vi "Vision Processing.vi"(4 "error in (no error)":errorcluster, 5 "Camera Type":enum16{"206", "1011"}(ring)=enum."1011", 6 "Camera Name":string="Camera") -> ()   [LabVIEW 2012]
uses:
  Robot Global Data.vi
  <vilib>/vision/NI_Vision_Development_Module.lvlib
panel:
  in  "Color Enabled":bool
  in  "Range":cluster{"Lower value":sgl, "Upper value":sgl}={"Lower value"=247.60869, "Upper value"=255.0} {"Lower value" scale=0.0..255.0; "Upper value" scale=0.0..255.0}
  out "Target Info":cluster{"X":dbl, "Y":dbl, "Distance (ft)":dbl}
  in  "Enable Vision":bool=TRUE
  in  "View":bool
  out "Target Info":T1(array[cluster])
  in  "Area Size Limit %":dbl=0.5
  in  "Particle Count Limit":i32=8
  in  "Score Limits":T2={"Rect Coverage"=60.0, "X Edge Strength"=40.0, "Y Edge Strength"=60.0, "Center"=75.0, "Outer"=75.0}
  in  "View":bool
  out "Processed Image":T3(plugin-control)
  out "Original Image":T3(plugin-control)
  # "Instructions:\nProcessing the reflective tape that is illuminated by a ring light can be based\non color or light intensity.\nParticles within the image are scored by rectangle coverage, aspect ratio, and\nfor being hollow with a bold edge. A particle is considered a target if all scores\nare above the score limits. Particles can be annotated -- surrounded by\na rectangle and scores drawn to the left .\nTo control the number of particles being scored, use the count limit and the size\nlimit."
  # "To debug, Enable using the View button.\nFor color processing, you can click in the image to select the color for processing."
  # "Enable by clicking the View button.\nGreen scores are above the limit, orange are below. Inner/outer rect\nindicates all passed."
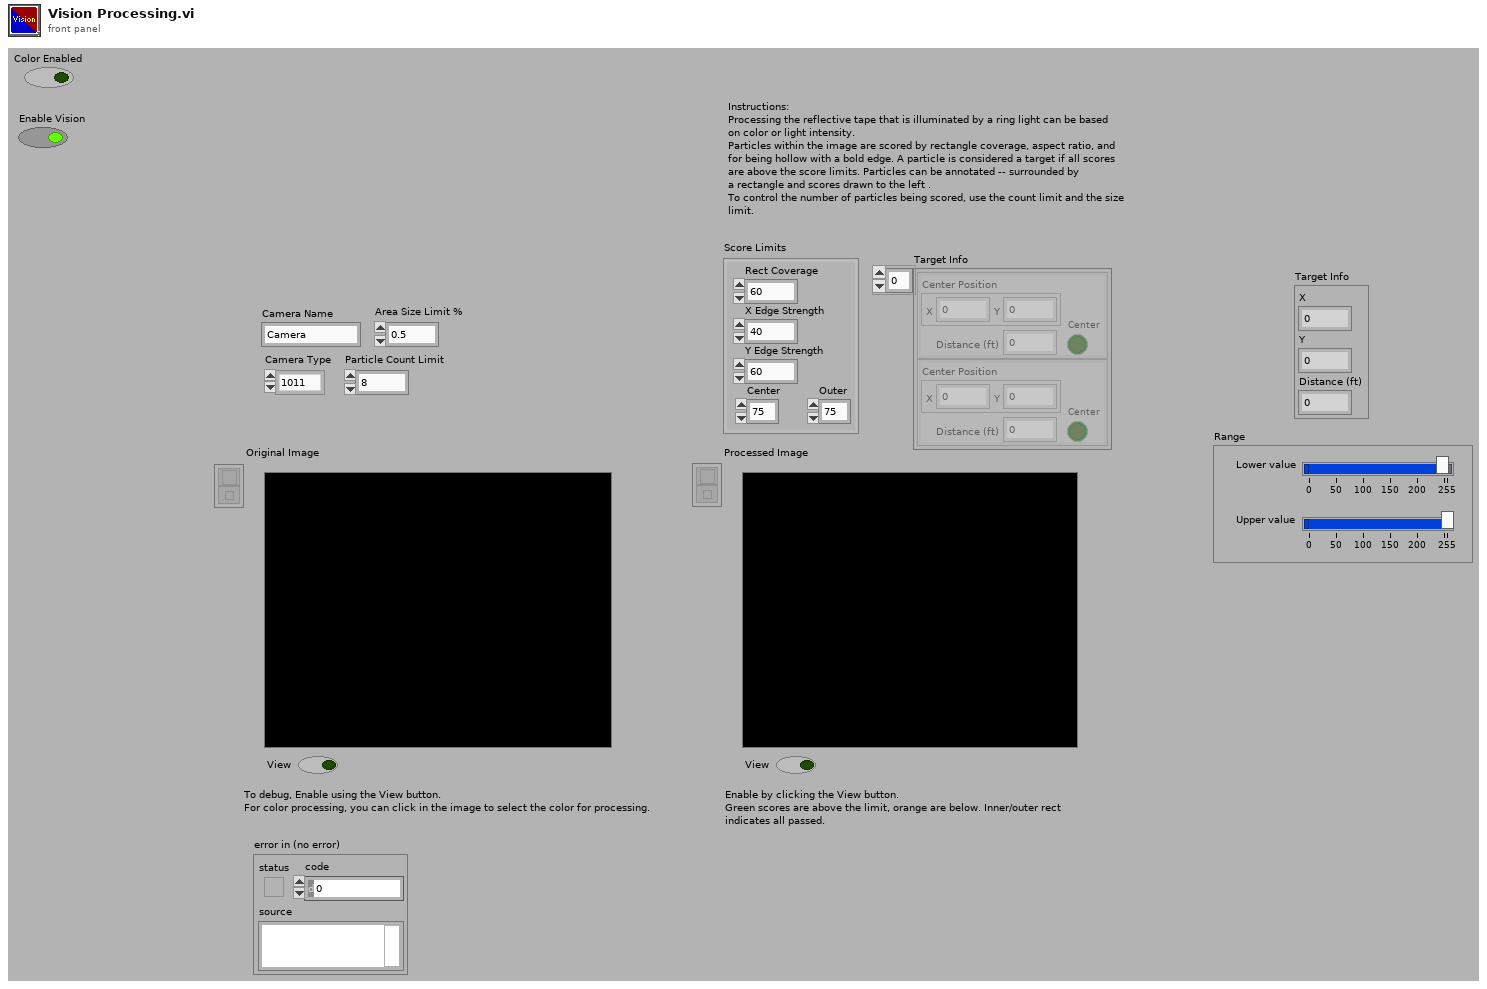
[diagram p1: front panel]
types:
  T1 = cluster{"Center Position":cluster{"X":dbl, "Y":dbl}, "Distance (ft)":dbl, "Center":bool}[]
  T2 = cluster{"Rect Coverage":dbl, "X Edge Strength":dbl, "Y Edge Strength":dbl, "Center":dbl, "Outer":dbl}
  T3 = typedef "IMAQ Image.ctl" = refnum<image>
  T4 = typedef "Image Type" = u32
  T5 = typedef "WPI_CameraDevRef.ctl" = cluster{"Camera Address":string, "CameraStatus":errorcluster, "Acquire Image Notifier":refnum<notifier>}
  T6 = cluster{"Position":cluster{"X":dbl, "Y":dbl}, "Distance (ft)":dbl, "Center":bool}[]
  T7 = typedef "WPI_CameraImageSize.ctl" = enum16{"640x480", "320x240", "160x120"}
  T8 = cluster{cluster{"Left":dbl, "Top":dbl, "Right":dbl, "Bottom":dbl}, "Scores":dbl[], cluster{"Long":dbl, "Short":dbl}}[]
  T9 = cluster{"Target Center (-1 to 1)":cluster{"X":dbl, "Y":dbl}, "Distance (ft)":dbl, "Center Target":bool}
  T10 = cluster{"Target Center (-1 to 1)":cluster{"X":dbl, "Y":dbl}, "Distance (ft)":dbl, "Center Target":bool}[]
  T11 = cluster{"Left":dbl, "Top":dbl, "Right":dbl, "Bottom":dbl}
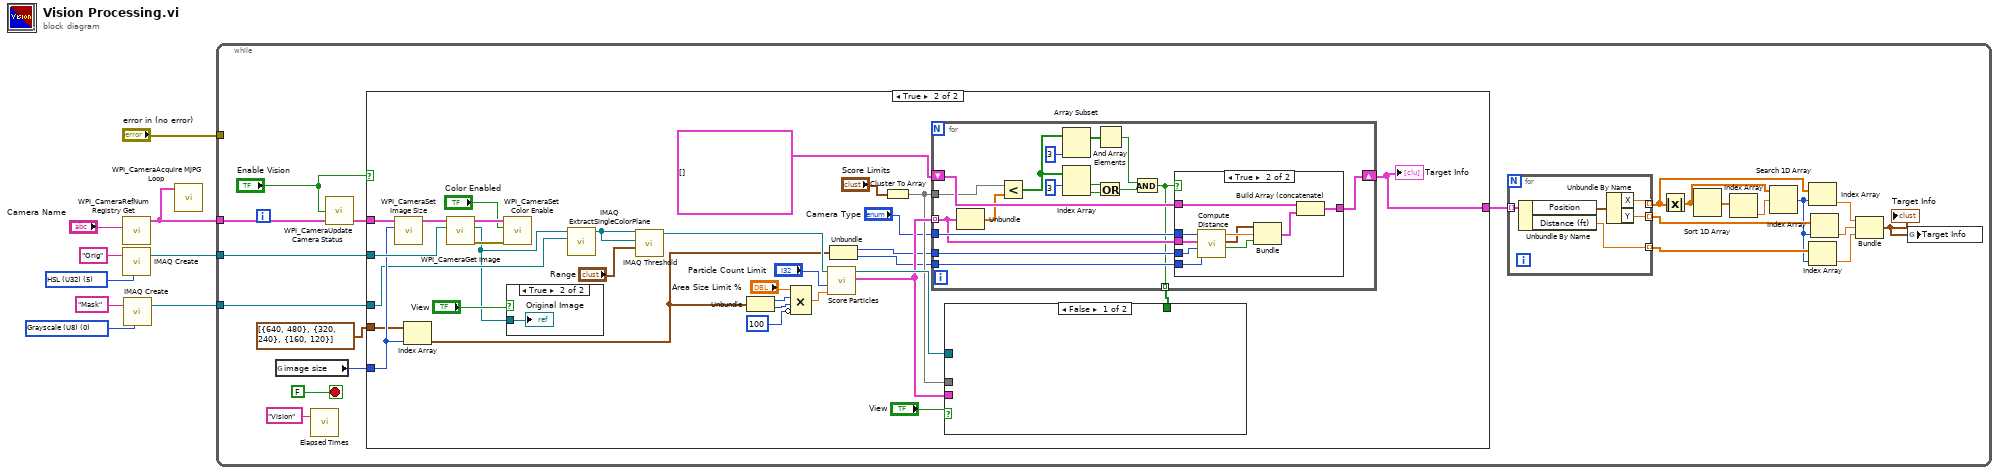
[diagram p0: block diagram]
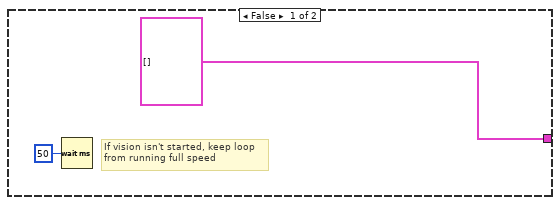
[diagram p2: hidden frame]
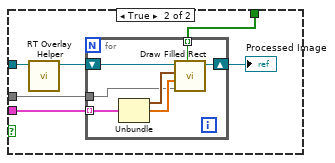
[diagram p4: hidden frame]
diagram:
  w3 = T4 0 items=["Grayscale (U8)", "Grayscale (I16)", "Grayscale (SGL)", "Complex (CSG)", "RGB (U32)", "HSL (U32)", "RGB (U64)", "Grayscale (U16)"] ("Image Type")
  w8 = T4 5 items=["Grayscale (U8)", "Grayscale (I16)", "Grayscale (SGL)", "Complex (CSG)", "RGB (U32)", "HSL (U32)", "RGB (U64)", "Grayscale (U16)"] ("Image Type")
  n1 = call <vilib>:"WPI_CameraRefNum Registry Get.vi"("refnum name"="Camera Name") -> ("CameraDevRef"=w5:T5)  [unwired: 9 in, 1 out]
  n2 = call "IMAQ Create"("Image Name"="Orig", "Image Type"=w8) -> ("New Image"=w7:T3)  [unwired: 2 in, 2 out]
  n3 = call "IMAQ Create"("Image Name"="Mask", "Image Type"=w3) -> ("New Image"=w1:T3)  [unwired: 2 in, 2 out]
  n4 = call <vilib>:"WPI_CameraAcquire MJPG Loop.vi"("CameraDevRef"=w5) -> ()  [unwired: 11 in]
  n5 = while {
    tunnel: w7 -> [w29]
    tunnel: w5 -> [w28]
    tunnel: "error in (no error)" -> [_]
    tunnel: w1 -> [w25]
    stop <- FALSE stop-if-true
    n6 = global read "Robot Global Data.vi" "image size"() -> (w26:T7)
    n7 = call "Elapsed Times.vi"("Call Name"="Vision") -> ()  [unwired: 2 in, 1 out]
    n8 = call <vilib>:"WPI_CameraUpdate Camera Status.vi"("CameraDevRef In"=w28, "Enable Vision"="Enable Vision") -> ("CameraDevRef Out"=w27:T5)  [unwired: 3 in]
    n9 = case shown="True" "Enable Vision" {
      tunnel: w29 -> [_ w64]
      tunnel: w27 -> [_ w60]
      tunnel: w26 -> [_ w57]
      tunnel: w25 -> [_ w53]
      tunnel: cluster{i32, i32}[] [{640, 480}, {320, 240}, {160, 120}] -> [_ w56]
      tunnel: [T6 [] w47] -> w21
      frame False {
        # "If vision isn't started, keep loop\nfrom running full speed"
        n10 = Wait (ms)(milliseconds to wait=u32 50) -> ()  [unwired: 1 out]
      }
      frame True {
        n11 = call <vilib>:"WPI_CameraSet Image Size.vi"("Image Size"=w57, "CameraDevRef"=w60) -> ("CameraDevRef Out"=w61:T5)  [unwired: 8 in, 1 out]
        n12 = Index Array(array=w56, index=w57) -> (element=w48:cluster{i32, i32})
        n13 = call <vilib>:"WPI_CameraGet Image.vi"("Image"=w64, "CameraDevRef"=w61) -> ("error out"=w62:errorcluster, "Image Out"=w52:T3, "CameraDevRef Out"=w63:T5)  [unwired: 7 in]
        n14 = call <vilib>:"WPI_CameraSet Color Enable.vi"("error in (no error)"=w62, "Color Enabled"="Color Enabled", "CameraDevRef"=w63) -> ()  [unwired: 7 in, 2 out]
        n15 = case shown="True" "View" {
          tunnel: w52 -> [_ w111]
          frame False {
          }
          frame True {
            "Original Image" <- w111
          }
        }
        n16 = call "IMAQ ExtractSingleColorPlane"("Image Dst"=w53, "Image Src"=w52) -> ("Image Dst Out"=w45:T3)  [unwired: 8 in, 1 out]
        n17 = call "IMAQ Threshold"("Range"="Range", "Image Dst"=w45, "Image Src"=w45) -> ("Image Dst Out"=w58:T3)  [unwired: 3 in, 5 out]
        n18 = Unbundle(w48) -> (w41:i32, w40:i32)
        n19 = Compound Arithmetic op=MULTIPLY("Area Size Limit %", w41, w40, invert 100 ("length")) -> (w38:dbl)
        n20 = call "Score Particles.vi"("Area Size Limit"=w38, "Particle Count Limit"="Particle Count Limit", "Image Refnum in"=w58) -> ("Scored Particle Info"=w67:T8, "Image Refnum out"=w69:T3)  [unwired: 7 in]
        n21 = Unbundle(w48) -> (w55:i32, w54:i32)
        n22 = Cluster To Array(cluster="Score Limits") -> (array=w65:dbl[])
        n23 = for {
          shift-right: [w85] -> w47
          shift-left: T6 [] -> [w86]
          tunnel: w55 -> [w84]
          tunnel: w67 -> [w79] mode=indexing
          tunnel: w65 -> [w81]
          tunnel: "Camera Type" -> [w83]
          tunnel: w54 -> [w80]
          tunnel: [w70] -> w49 mode=indexing
          n24 = Unbundle(w79) -> ("Scores"=w82:dbl[])  [unwired: 2 out]
          n25 = Less?(x=w81, y=w82) -> (x < y?=w71:bool[])
          n26 = Array Subset(array=w71, length=3) -> (w73:bool[])  [unwired: 1 in]
          n27 = Index Array(array=w71, index #1=3 ("length")) -> (element #1=w75:bool, element #2=w76:bool)  [unwired: 1 in]
          n28 = And Array Elements(Boolean array=w73) -> (logical AND=w78:bool)
          n29 = Or(x=w75, y=w76) -> (x .or. y?=w77:bool)
          n30 = And(x=w78, y=w77) -> (x .and. y?=w70:bool)
          n31 = case shown="True" w70 {
            tunnel: w86 -> [w87 w97]
            tunnel: [w87 w96] -> w85
            tunnel: w84 -> [_ w94]
            tunnel: w83 -> [_ w92]
            tunnel: w80 -> [_ w91]
            tunnel: w79 -> [_ w89]
            frame False {
            }
            frame True {
              n32 = call "Compute Distance.vi"("Y Image Resolution"=w91, "X Image Resolution"=w94, "Particle Scores"=w89, "Camera Type"=w92) -> ("Center Target"=w88:bool, "Target Center (-1 to 1)"=w90:cluster{"X":dbl, "Y":dbl}, "Distance (ft)"=w93:dbl)  [unwired: 5 in]
              n33 = Bundle("Target Center (-1 to 1)"=w90, "Distance (ft)"=w93, "Center Target"=w88) -> (w95:T9)  [unwired: 1 in]
              n34 = Build Array (concatenate)(w97, w95) -> (w96:T10)
            }
          }
        }
        "Target Info" <- w47
        n35 = case shown="False" "View" {
          tunnel: w69 -> [_ w100]
          tunnel: w67 -> [_ w102]
          tunnel: w65 -> [_ w101]
          tunnel: w49 -> [_ w98]
          frame False {
          }
          frame True {
            n36 = call "RT Overlay Helper.vi"("Refnum in"=w100) -> ("Refnum out"=w103:T3)  [unwired: 10 in]
            n37 = for {
              shift-right: [w109] -> w99
              shift-left: w103 -> [w110]
              tunnel: w102 -> [w106] mode=indexing
              tunnel: w101 -> [w105]
              tunnel: w98 -> [w104] mode=indexing
              n38 = Unbundle(w106) -> (w107:T11, "Scores"=w108:dbl[])  [unwired: 1 out]
              n39 = call "Draw Filled Rect.vi"("Limit Passed"=w104, "Limits"=w105, "Scores"=w108, "Bounding Box"=w107, "image in"=w110) -> ("image out"=w109:T3)  [unwired: 6 in]
            }
            "Processed Image" <- w99
          }
        }
      }
    }
    n40 = for {
      tunnel: w21 -> [w35] mode=indexing
      tunnel: [w33] -> w17 mode=indexing
      tunnel: [w32] -> w16 mode=indexing
      tunnel: [w31] -> w15 mode=indexing
      n41 = Unbundle By Name(w35) -> ("Position"=w34:cluster{"X":dbl, "Y":dbl}, "Distance (ft)"=w31:dbl)
      n42 = Unbundle By Name(w34) -> ("X"=w33:dbl, "Y"=w32:dbl)
    }
    n43 = Absolute Value(x=w17) -> (abs(x)=w19:dbl[])
    n44 = Sort 1D Array(array=w19) -> (sorted array=w20:dbl[])
    n45 = Index Array(array=w20) -> (element=w18:dbl)  [unwired: 1 in]
    n46 = Search 1D Array(1D array=w19, element=w18) -> (index of element=w14:i32)  [unwired: 1 in]
    n47 = Index Array(array=w17, index=w14) -> (element=w13:dbl)
    n48 = Index Array(array=w15, index=w14) -> (element=w11:dbl)
    n49 = Index Array(array=w16, index=w14) -> (element=w12:dbl)
    n50 = Bundle("X"=w13, "Y"=w12, "Distance (ft)"=w11) -> (w10:cluster{"X":dbl, "Y":dbl, "Distance (ft)":dbl})  [unwired: 1 in]
    "Target Info" <- w10
    n51 = global write "Robot Global Data.vi" "Target Info"(w10) -> ()
  }
